vi "Choreo_SwerveSample_Pack.vi"(9 "ChoreoSwerveSample":T1, 11 "RawData":u8[](array[numeric])) -> (3 "RawData Out":u8[](array[numeric]))   [LabVIEW 2019, in "ChoreoLib.lvlib"]
doc: "Constructs a SwerveSample with the specified parameters.\n\n */\n\nInputs: \n - t - double - The timestamp of this sample, relative to the beginning of the trajectory.\n - x - double - The X position of the sample in meters.\n - y - double - The Y position of the sample in meters.\n - heading - double - The heading of the sample in radians, with 0 being in the +X direction.\n - vx - double - The velocity of the sample in the X direction in m/s.\n - vy - double - The velocity of the sample in the Y direction in m/s.\n - omega - double - The angular velocity of the sample in rad/s.\n - ax - double - The acceleration of the sample in the X direction in m/s².\n - ay - double - The acceleration of the sample in the Y direction in m/s².\n - alpha - double - The angular acceleration of the sample in rad/s².\n - moduleForcesX - double array - The force on each swerve module in the X direction in Newtons. Module forces appear in the following order: [FL, FR, BL, BR].\n - moduleForcesY - double array - The force on each swerve module in the Y direction in Newtons. Module forces appear in the following order: [FL, FR, BL, BR].\n\nOutputs:\n - ChoreoSwerveSample - cluster - Cluster containing sample data"
uses:
  TypeDef/ChoreoSwerveSample.ctl
  ChoreoLib.lvlib
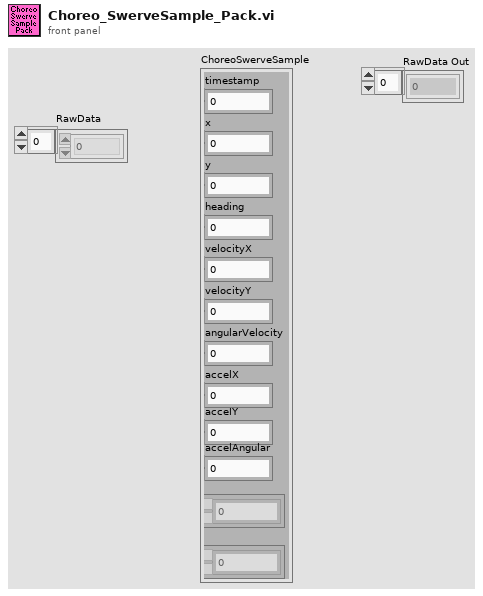
[diagram p1: front panel]
types:
  T1 = typedef "ChoreoLib.lvlib/ChoreoSwerveSample.ctl" = cluster{"timestamp":dbl, "x":dbl, "y":dbl, "heading":dbl, "velocityX":dbl, "velocityY":dbl, "angularVelocity":dbl, "accelY":dbl, "accelX":dbl, "accelAngular":dbl, "forceX":dbl[], "forceY":dbl[]}
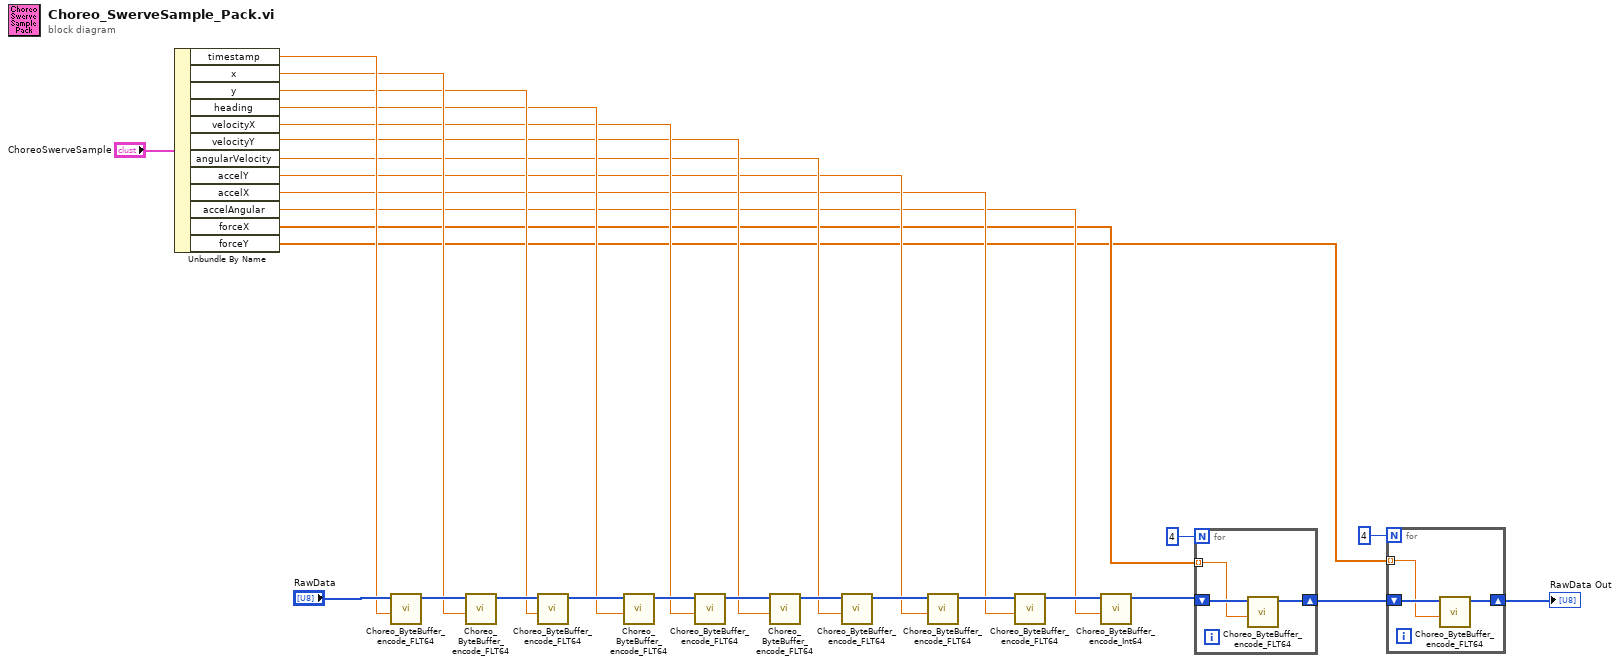
[diagram p0: block diagram]
diagram:
  n1 = Unbundle By Name("ChoreoSwerveSample") -> ("timestamp"=w21:dbl, "x"=w20:dbl, "y"=w19:dbl, "heading"=w9:dbl, "velocityX"=w8:dbl, "velocityY"=w7:dbl, "angularVelocity"=w6:dbl, "accelY"=w5:dbl, "accelX"=w4:dbl, "accelAngular"=w3:dbl, "forceX"=w2:dbl[], "forceY"=w1:dbl[])
  n2 = call "Choreo_ByteBuffer_encode_FLT64.vi"("FLT64_Value"=w21, "RawData In"="RawData") -> ("RawData Out"=w23:u8[])  [unwired: 9 in]
  n3 = call "Choreo_ByteBuffer_encode_FLT64.vi"("FLT64_Value"=w20, "RawData In"=w23) -> ("RawData Out"=w22:u8[])  [unwired: 9 in]
  n4 = call "Choreo_ByteBuffer_encode_FLT64.vi"("FLT64_Value"=w19, "RawData In"=w22) -> ("RawData Out"=w18:u8[])  [unwired: 9 in]
  n5 = call "Choreo_ByteBuffer_encode_FLT64.vi"("FLT64_Value"=w9, "RawData In"=w18) -> ("RawData Out"=w17:u8[])  [unwired: 9 in]
  n6 = call "Choreo_ByteBuffer_encode_FLT64.vi"("FLT64_Value"=w8, "RawData In"=w17) -> ("RawData Out"=w16:u8[])  [unwired: 9 in]
  n7 = call "Choreo_ByteBuffer_encode_FLT64.vi"("FLT64_Value"=w7, "RawData In"=w16) -> ("RawData Out"=w15:u8[])  [unwired: 9 in]
  n8 = call "Choreo_ByteBuffer_encode_FLT64.vi"("FLT64_Value"=w6, "RawData In"=w15) -> ("RawData Out"=w14:u8[])  [unwired: 9 in]
  n9 = call "Choreo_ByteBuffer_encode_FLT64.vi"("FLT64_Value"=w5, "RawData In"=w14) -> ("RawData Out"=w13:u8[])  [unwired: 9 in]
  n10 = call "Choreo_ByteBuffer_encode_FLT64.vi"("FLT64_Value"=w4, "RawData In"=w13) -> ("RawData Out"=w12:u8[])  [unwired: 9 in]
  n11 = call "Choreo_ByteBuffer_encode_Int64.vi"("Int64_Value"=w3, "RawData In"=w12) -> ("RawData Out"=w11:u8[])  [unwired: 9 in]
  n12 = for {
    N: 4 -> [_]
    shift-right: [w31] -> w25
    shift-left: w11 -> [w30]
    tunnel: w2 -> [w29] mode=indexing
    n13 = call "Choreo_ByteBuffer_encode_FLT64.vi"("FLT64_Value"=w29, "RawData In"=w30) -> ("RawData Out"=w31:u8[])  [unwired: 9 in]
  }
  n14 = for {
    N: 4 -> [_]
    shift-right: [w34] -> w10
    shift-left: w25 -> [w33]
    tunnel: w1 -> [w32] mode=indexing
    n15 = call "Choreo_ByteBuffer_encode_FLT64.vi"("FLT64_Value"=w32, "RawData In"=w33) -> ("RawData Out"=w34:u8[])  [unwired: 9 in]
  }
  "RawData Out" <- w10
